vi "FP_recorder.vi"() -> ()   [LabVIEW 2013]
uses:
  <userlib>/caLab/Private/Get_PV.vi
panel:
  out "Cluster":T1
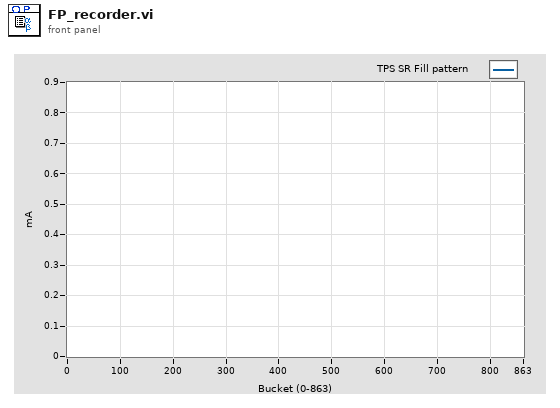
[diagram p1: front panel]
types:
  T1 = cluster{"SR Fill pattern":dbl[], "date/time string":string}
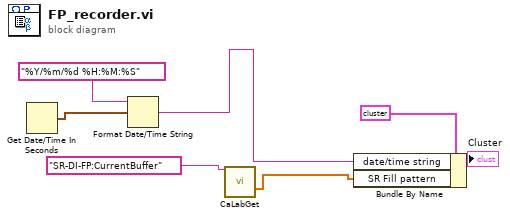
[diagram p0: block diagram]
diagram:
  n1 = Get Date/Time In Seconds() -> (seconds since 1Jan1904=w6:timestamp)
  n2 = Format Date/Time String(time format string (%c)="%Y/%m/%d %H:%M:%S", seconds (now)=w6) -> (date/time string=w2:string)  [unwired: 1 in]
  n3 = call-poly <userlib>:"CaLabGet.vi"("PV Name"="SR-DI-FP:CurrentBuffer") -> ("Value Array (number)"=w1:dbl[])  [unwired: 8 in, 6 out]
  n4 = Bundle By Name(cluster=T1 {"SR Fill pattern"=array[864 elements], "date/time string"=""} ("Cluster"), "date/time string"=w2, "SR Fill pattern"=w1) -> (→"Cluster":T1)
